vi "RoiName.vi"(10 "Image":T2, 11 "ROI":T3) -> (2 "Imageout":T2)   [LabVIEW 2015]
uses:
  <vilib>/vision/Image Controls.llb/IMAQ Image.ctl
panel:
  in  "Font, Size & Style":T1={"Desired Font (Application)"=enum."Application Font", "[User-specified Font]"={"Font Name"="", "Size"=33, "Strikeout?"=FALSE, "Italic?"=FALSE, "Underline?"=FALSE, "Outline?"=FALSE, "Shadow?"=FALSE, "Bold?"=FALSE, "Rotation Angle"=0.0}, "Horizontal Alignment"=0, "Vertical Alignment"=0} {"Horizontal Alignment" items=["Left", "Center", "Right"]; "Vertical Alignment" items=["Bottom", "Top", "Baseline"]}
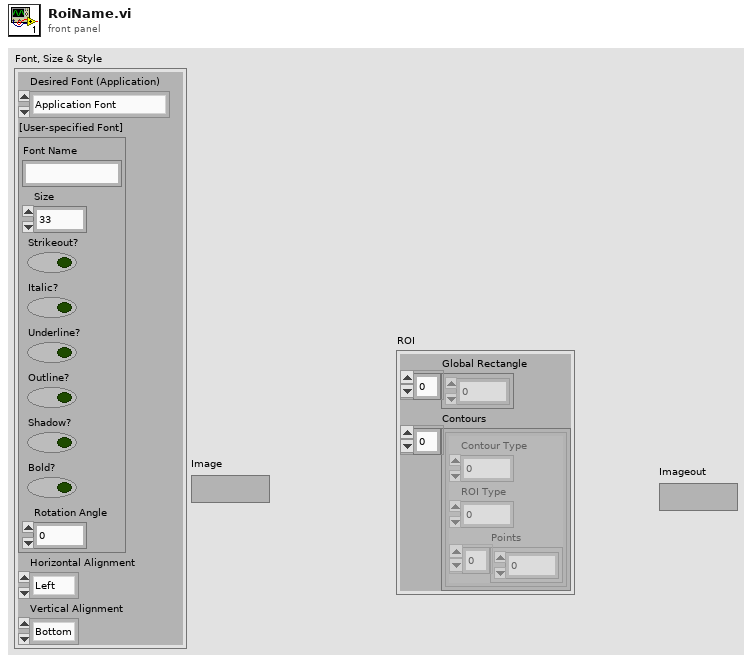
[diagram p1: front panel]
types:
  T1 = cluster{"Desired Font (Application)":enum16{"User-specified Font", "Application Font", "System Font", "Dialog Font"}, "[User-specified Font]":cluster{"Font Name":string, "Size":i16, "Strikeout?":bool, "Italic?":bool, "Underline?":bool, "Outline?":bool, "Shadow?":bool, "Bold?":bool, "Rotation Angle":dbl}, "Horizontal Alignment":i16, "Vertical Alignment":i16}
  T2 = typedef "IMAQ Image.ctl" = refnum<image>
  T3 = cluster{"Global Rectangle":i32[], "Contours":cluster{"Contour Type":u32, "ROI Type":u32, "Points":i32[]}[]}
  T4 = cluster{"Contour Type":u32, "ROI Type":u32, "Points":i32[]}[]
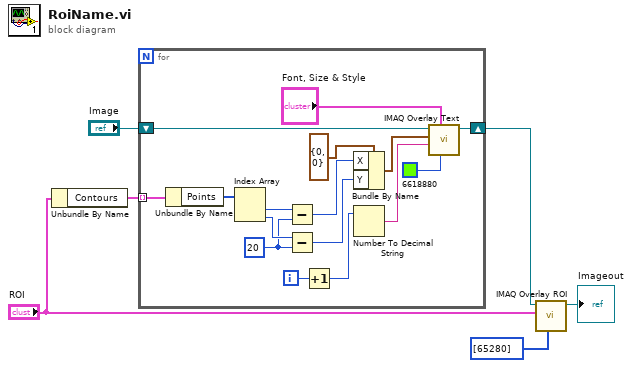
[diagram p0: block diagram]
diagram:
  n1 = Unbundle By Name("ROI") -> ("Contours"=w6:T4)
  n2 = for {
    shift-right: [w7] -> w4
    shift-left: "Image" -> [w13]
    tunnel: w6 -> [w22] mode=indexing
    i -> [w11]
    w17 = 20 ("y")
    n3 = Unbundle By Name(w22) -> ("Points"=w21:i32[])
    n4 = Index Array(array=w21) -> (element #1=w19:i32, element #2=w18:i32)  [unwired: 2 in]
    n5 = Subtract(x=w19, y=w17) -> (x-y=w16:i32)
    n6 = Subtract(x=w18, y=w17) -> (x-y=w15:i32)
    n7 = Increment(x=w11) -> (x+1=w10:i32)
    n8 = Bundle By Name(cluster=cluster{"X":i32, "Y":i32} {"X"=0, "Y"=0} ("Origin"), "X"=w16, "Y"=w15) -> (w14:cluster{"X":i32, "Y":i32})
    n9 = Number To Decimal String(number=w10) -> (decimal integer string=w9:string)  [unwired: 1 in]
    n10 = call "IMAQ Overlay Text"("Text Color (black)"=u32 6618880, "Font, Size & Style"="Font, Size & Style", "String"=w9, "Origin"=w14, "Image"=w13) -> ("Image Out"=w7:T2)  [unwired: 5 in, 1 out]
  }
  n11 = call "IMAQ Overlay ROI"("Colors (Green)"=u32[] [65280], "ROI Descriptor"="ROI", "Image"=w4) -> ("Image Out"=→"Imageout":T2)  [unwired: 7 in, 1 out]
